vi "Convert PID Gains.vi"   [LabVIEW 2017]
doc: "Converts PID gains in the Academic, Parallel, or Series form to the normalized Parallel form that the PID VI expects."
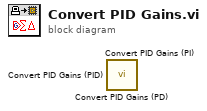
[diagram p0: block diagram]
diagram:
  n1 = call <vilib>:"Convert PID Gains (PD).vi"() -> ()  [unwired: 14 in, 2 out]
  n2 = call <vilib>:"Convert PID Gains (PI).vi"() -> ()  [unwired: 14 in, 2 out]
  n3 = call <vilib>:"Convert PID Gains (PID).vi"() -> ()  [unwired: 14 in, 2 out]
